vi "Write.vi"(8 "error in":errorcluster, 10 "Command":string="*IDN?", 11 "Serial in":refnum<class "Serial.lvclass">) -> (0 "error out":errorcluster, 3 "Serial out":refnum<class "Serial.lvclass">)   [LabVIEW 2019, in "Serial.lvlib" / "Serial.lvclass"]
uses:
  Serial.lvclass
  Serial.lvclass/Serial.ctl
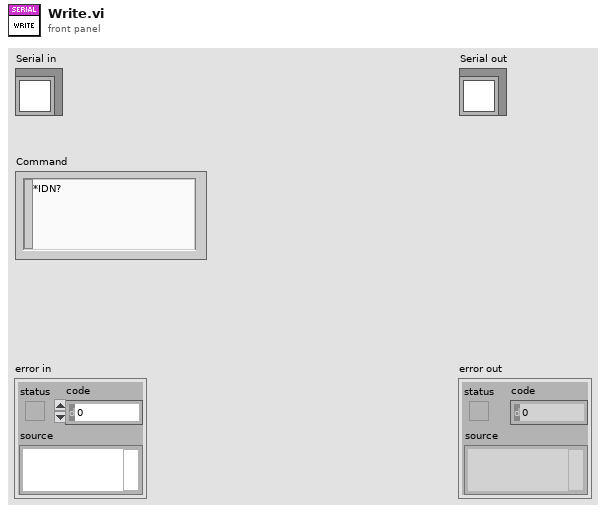
[diagram p1: front panel]
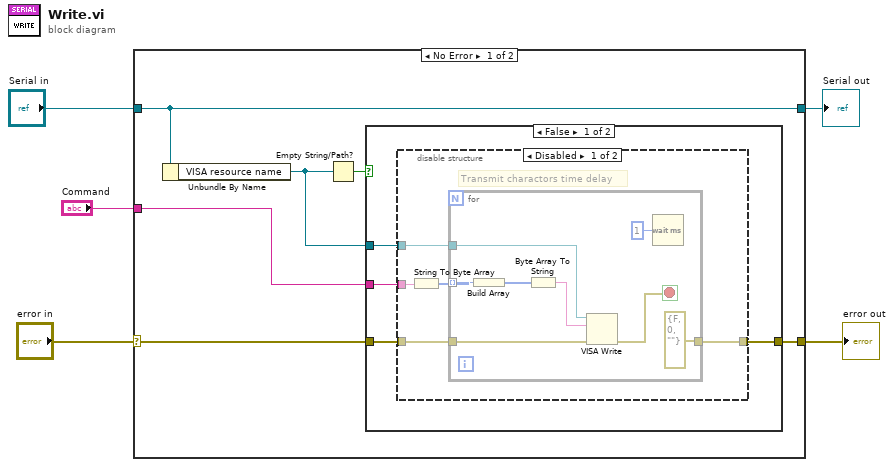
[diagram p0: block diagram]
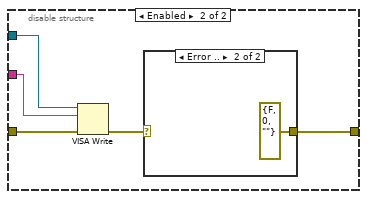
[diagram p2: hidden frame]
diagram:
  n1 = case shown="No Error" "error in" {
    selector: "error in" -> [w10 w38]
    tunnel: [w9 w38] -> w4
    tunnel: [w11 w37] -> w2
    tunnel: "Serial in" -> [w11 w37]
    tunnel: "Command" -> [w8 _]
    frame No Error {
      n2 = Unbundle By Name(w11) -> ("VISA resource name"=w7:refnum<visa-resource-name>)
      n3 = Empty String/Path?(string/path=w7) -> (empty?=w6:bool)
      n4 = case shown="False" w6 {
        tunnel: w10 -> [w15 w36]
        tunnel: [w14 w36] -> w9
        tunnel: w8 -> [w13 _]
        tunnel: w7 -> [w12 _]
        frame False {
          n5 = disable-structure shown="Disabled" {
            disable-tunnel: w15 -> [w19 w32]
            disable-tunnel: [w18 w31] -> w14
            disable-tunnel: w13 -> [w17 w30]
            disable-tunnel: w12 -> [w16 w29]
            frame Disabled {
              # "Transmit charactors time delay"
              n6 = String To Byte Array(string=w17) -> (unsigned byte array=w20:u8[])
              n7 = for {
                tunnel: w20 -> [w27] mode=indexing
                tunnel: w16 -> [w24]
                tunnel: w19 -> [w28]
                tunnel: [errorcluster {"status"=FALSE, "code"=0, "source"=""} ("error out")] -> w18
                stop <- w22 stop-if-true
                n8 = Build Array(w27) -> (w26:u8[])
                n9 = Byte Array To String(unsigned byte array=w26) -> (string=w25:string)
                n10 = VISA Write(VISA resource name=w24, write buffer=w25, error in (no error)=w28) -> (error out=w22:errorcluster)  [unwired: 2 out]
                n11 = Wait (ms)(milliseconds to wait=u32 1) -> ()  [unwired: 1 out]
              }
            }
            frame Enabled {
              n12 = VISA Write(VISA resource name=w29, write buffer=w30, error in (no error)=w32) -> (error out=w33:errorcluster)  [unwired: 2 out]
              n13 = case shown="Error .." w33 {
                selector: w33 -> [w34 _]
                tunnel: [w34 errorcluster {"status"=FALSE, "code"=0, "source"=""} ("error IO")] -> w31
                frame No Error {
                }
                frame Error {
                }
              }
            }
          }
        }
        frame True {
        }
      }
    }
    frame Error {
    }
  }
  "error out" <- w4
  "Serial out" <- w2
